vi "AppConfig.vi"(8 "error in (no error)":errorcluster, 11 "LSEPlugin":refnum<class "LSEPlugin.lvclass">) -> (0 "error out":errorcluster, 3 "LSEPlugin out":refnum<class "LSEPlugin.lvclass">)   [LabVIEW 2014, in "AppPlugins.lvlib" / "LSEPlugin.lvclass"]
uses:
  LSEPlugin.lvclass
  LSEPlugin.lvclass/LSEPlugin.ctl
  Accessors/Read LSEConfig.vi
  Accessors/Write LSEConfig.vi
panel:
  in  "Least Square\nNoiseVariance":dbl=0.001
  in  "Save Button":bool
  in  "Cancel Button 2":bool
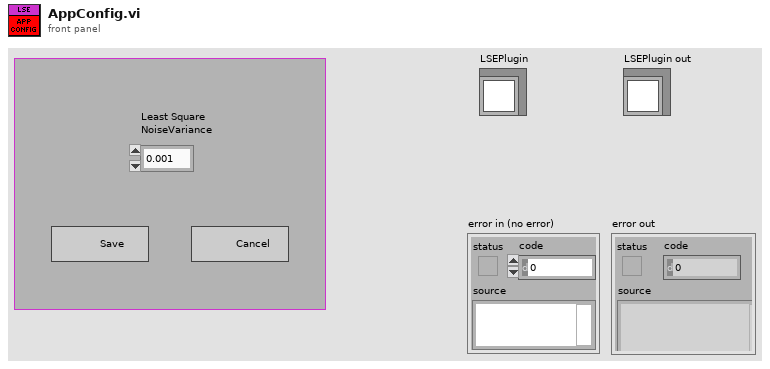
[diagram p1: front panel]
types:
  T1 = typedef "AppPlugins.lvlib/LSEPlugin.lvclass/LSEConfig.ctl" = cluster{"NoiseVariance":dbl, "IEEESystem":u32, "PMULocations":u32[], "Vindex":i32, "Iindex":i32, "DynamicRef":string}
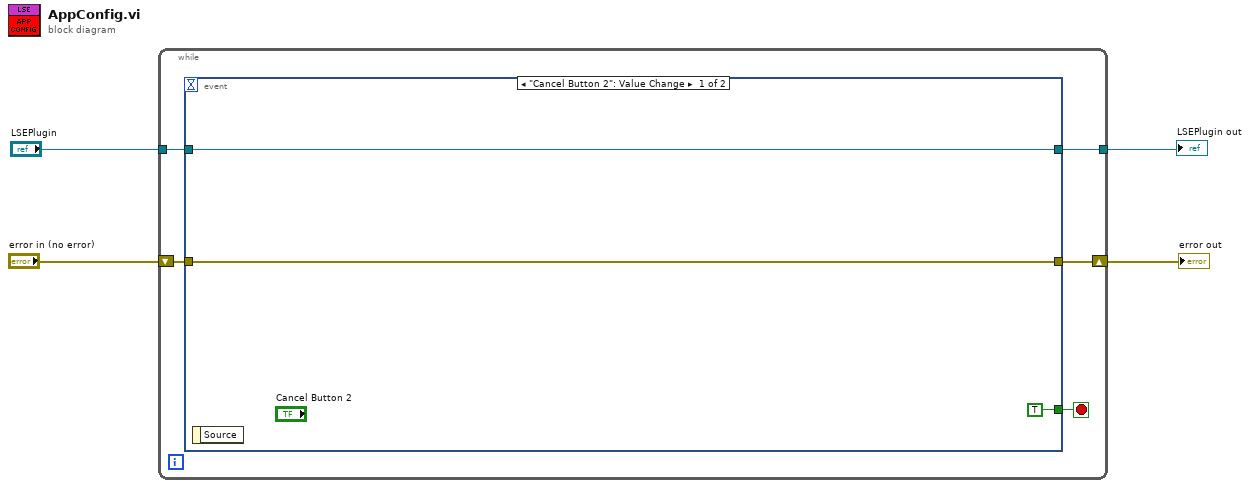
[diagram p0: block diagram]
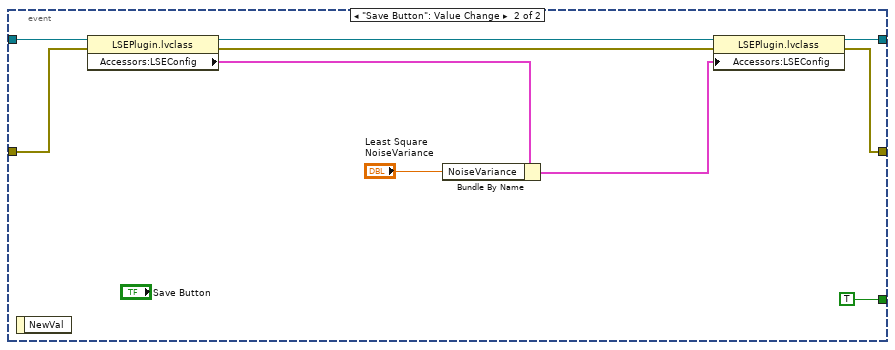
[diagram p2: hidden frame]
diagram:
  n1 = while {
    shift-right: [w9] -> w3
    shift-left: "error in (no error)" -> [w7]
    tunnel: [w8] -> w4
    tunnel: "LSEPlugin" -> [w5]
    stop <- w6 stop-if-true
    n2 = event shown="[0] \"Cancel Button 2\": Value Change" {
      selector: _ -> [_ _]
      dyn-events: _ -> [_ _]
      timeout: _ -> [_ _]
      tunnel: [w12 w22] -> w9
      tunnel: [w10 w21] -> w8
      tunnel: w7 -> [w12 w18]
      tunnel: [TRUE TRUE] -> w6
      tunnel: w5 -> [w10 w13]
      event "Cancel Button 2": Value Change {
        n3 = event-data() -> ()  [unwired: 1 in, 1 out]
      }
      event "Save Button": Value Change {
        n4 = event-data() -> ()  [unwired: 1 in, 1 out]
        n5 = property class="LSEPlugin.lvclass"(reference=w13, error in=w18) -> (reference out=w19:refnum<class "LSEPlugin.lvclass">, error out=w17:errorcluster, "Accessors:LSEConfig"=w16:T1)
        n6 = Bundle By Name(cluster=w16, "NoiseVariance"="Least Square\nNoiseVariance") -> (w14:T1)
        n7 = property class="LSEPlugin.lvclass"(reference=w19, error in=w17, "Accessors:LSEConfig"=w14) -> (reference out=w21:refnum<class "LSEPlugin.lvclass">, error out=w22:errorcluster)
      }
    }
  }
  "error out" <- w3
  "LSEPlugin out" <- w4
